vi "Speaker Cal.vi"(8 "error in":errorcluster, 9 "SEQ in":refnum<class "SEQ.lvclass">, 10 "Plow":dbl, 11 "P Cal Builder in":refnum<class "P Cal Builder.lvclass">) -> (0 "error out":errorcluster, 2 "SEQ out":refnum<class "SEQ.lvclass">, 3 "P Cal Builder out":refnum<class "P Cal Builder.lvclass">)   [LabVIEW 2015, in "P Cal Builder.lvclass"]
uses:
  P Cal Builder.lvclass
  Reusable/Sequence/SEQ/SEQ.lvclass
  Sequence/Set Pressure/Set Pressure.lvclass
  Reusable/Sequence/STEPS/LEAVES/String/String STEP.lvclass
  Calibration/Change Spk Pos/Change Speaker Position.lvclass
  Calibration/Wait/Wait.lvclass
  P Cal Builder.lvclass/P Cal Builder.ctl
  Reusable/Sequence/STEPS/LEAVES/String/String STEP.lvclass/String STEP.ctl
  Reusable/Sequence/STEPS/LEAVES/Double/Switch DBL.lvclass/Switch DBL.ctl
  Calibration/Wait/Wait.lvclass/Wait.ctl
  Reusable/Sequence/STEPS/LEAVES/Double/Switch DBL.lvclass
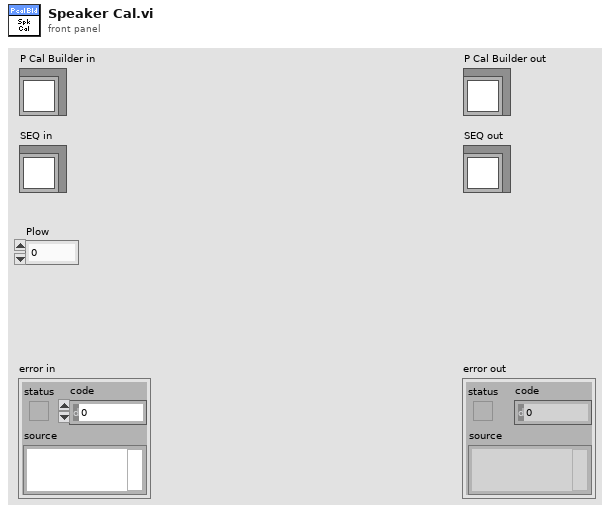
[diagram p1: front panel]
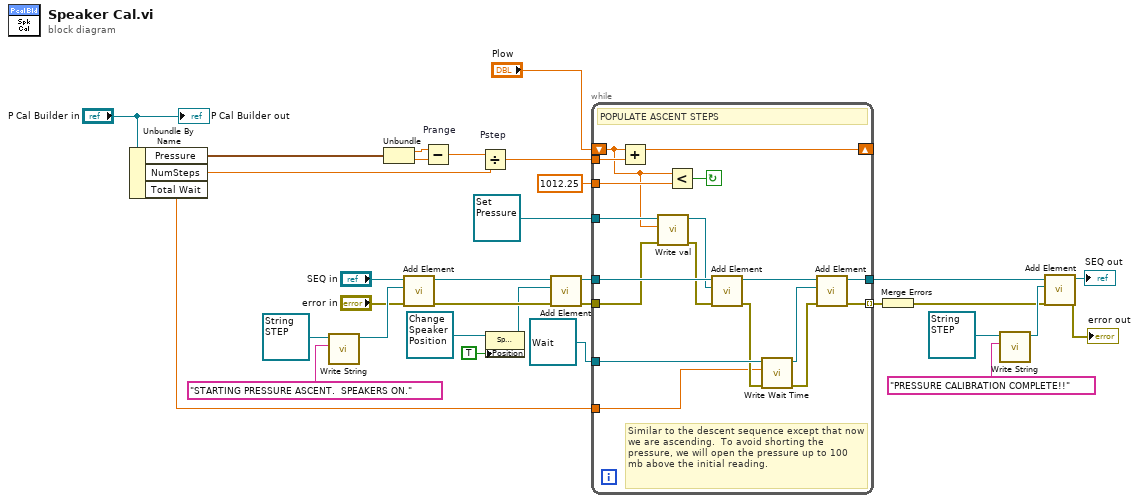
[diagram p0: block diagram]
diagram:
  n1 = Unbundle By Name("P Cal Builder in") -> ("Pressure"=w14:cluster{"Start":dbl, "Final":dbl}, "NumSteps"=w11:dbl, "Total Wait"=w6:dbl)
  n2 = call "Write String.vi"("String"="STARTING PRESSURE ASCENT.  SPEAKERS ON.", "String STEP in"=refnum<class "String STEP.lvclass"> refnum ("Std MSG STEP")) -> ("String STEP out"=w29:refnum<class "String STEP.lvclass">)  [unwired: 8 in, 1 out]
  n3 = Unbundle(w14) -> ("Start"=w9:dbl, "Final"=w13:dbl)
  n4 = call "Add Element.vi"("error in"="error in", "STEP"=w29, "SEQ in"="SEQ in") -> ("error out"=w20:errorcluster, "SEQ out"=w23:refnum<class "SEQ.lvclass">)  [unwired: 7 in]
  n5 = Subtract "Prange"(x=w9, y=w13) -> (x-y=w12:dbl)
  n6 = Divide "Pstep"(x=w12, y=w11) -> (x/y=w8:dbl)
  n7 = property class="Spk Pos"(reference=refnum<class "Change Speaker Position.lvclass"> refnum ("Spk Pos"), "Position"=TRUE) -> (reference out=w17:refnum<class "Change Speaker Position.lvclass">)  [unwired: 1 in, 1 out]
  n8 = call "Add Element.vi"("error in"=w20, "STEP"=w17, "SEQ in"=w23) -> ("error out"=w21:errorcluster, "SEQ out"=w22:refnum<class "SEQ.lvclass">)  [unwired: 7 in]
  n9 = while {
    tunnel: refnum<class "Set Pressure.lvclass"> refnum ("Set Pressure Step") -> [w46]
    tunnel: 1012.25 -> [w49]
    tunnel: w8 -> [w50]
    shift-right: [w45] -> _
    shift-left: "Plow" -> [w33]
    tunnel: w22 -> [w47]
    tunnel: refnum<class "Wait.lvclass"> refnum ("Wait") -> [w42]
    tunnel: [w37] -> w28
    tunnel: [w36] -> w31 mode=indexing
    tunnel: w21 -> [w35]
    tunnel: w6 -> [w34]
    stop <- w48 continue-if-true
    # "Similar to the descent sequence except that now we are ascending.  To avoid shorting the pressure, we will open the pressure up to 100 mb above the initial reading."
    # "POPULATE ASCENT STEPS"
    n10 = Add(x=w33, y=w50) -> (x+y=w45:dbl)
    n11 = call "Write val.vi"("error in (no error)"=w35, "val"=w33, "Switch DBL in"=w46) -> ("error out"=w44:errorcluster, "Switch DBL out"=w43:refnum<class "Set Pressure.lvclass">)  [unwired: 7 in]
    n12 = Less?(x=w33, y=w49) -> (x < y?=w48:bool)
    n13 = call "Add Element.vi"("error in"=w44, "STEP"=w43, "SEQ in"=w47) -> ("error out"=w40:errorcluster, "SEQ out"=w41:refnum<class "SEQ.lvclass">)  [unwired: 7 in]
    n14 = call "Write Wait Time.vi"("error in (no error)"=w40, "Wait Time"=w34, "Wait in"=w42) -> ("error out"=w39:errorcluster, "Wait out"=w38:refnum<class "Wait.lvclass">)  [unwired: 7 in]
    n15 = call "Add Element.vi"("error in"=w39, "STEP"=w38, "SEQ in"=w41) -> ("error out"=w36:errorcluster, "SEQ out"=w37:refnum<class "SEQ.lvclass">)  [unwired: 7 in]
  }
  n16 = Merge Errors(w31) -> (w24:errorcluster)
  n17 = call "Write String.vi"("String"="PRESSURE CALIBRATION COMPLETE!!", "String STEP in"=refnum<class "String STEP.lvclass"> refnum ("Std MSG STEP")) -> ("String STEP out"=w25:refnum<class "String STEP.lvclass">)  [unwired: 8 in, 1 out]
  n18 = call "Add Element.vi"("error in"=w24, "STEP"=w25, "SEQ in"=w28) -> ("error out"=→"error out":errorcluster, "SEQ out"=→"SEQ out":refnum<class "SEQ.lvclass">)  [unwired: 7 in]
  "P Cal Builder out" <- "P Cal Builder in"
